vi "TrALEX_NRG.vi"(0 "Analog Amplitude":dbl=1.0 format="%0.2p", 1 "Repetition Frequency":dbl=2.0 format="%.6f") -> ()   [LabVIEW 2011]
uses:
  <vilib>/DAQmx/write.llb/DAQmx Write (Analog Wfm 1Chan NSamp).vi
  <vilib>/DAQmx/create/channels.llb/DAQmx Create Channel (AO-Voltage-Basic).vi
  <vilib>/DAQmx/configure/timing.llb/DAQmx Timing (Sample Clock).vi
  <vilib>/DAQmx/create/channels.llb/DAQmx Create Channel (CO-Pulse Generation-Frequency).vi
  <vilib>/DAQmx/configure/events/hardwareSignals.llb/DAQmx Export Signal (Most Signals).vi
  <vilib>/DAQmx/configure/trigger.llb/DAQmx Start Trigger (Digital Edge).vi
  <vilib>/DAQmx/configure/timing.llb/DAQmx Timing (Implicit).vi
  <vilib>/DAQmx/miscellaneous.llb/DAQmx Fill In Error Info.vi
  <vilib>/measure/NI_MABase.lvlib
panel:
  in  "Three Colour Duty Cycle":dbl=0.3333333333333333 format="%.6f"
  in  "Stop Button":bool
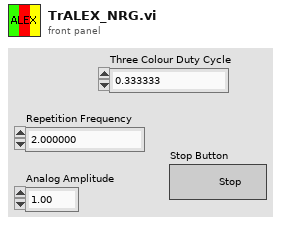
[diagram p1: front panel]
types:
  T1 = enum16{"Sine Wave", "Triangle Wave", "Square Wave", "Sawtooth Wave"}
  T2 = cluster{"Ao0 Sample Clock Rate":dbl, "Ao0 Sample Clock Rate":dbl}
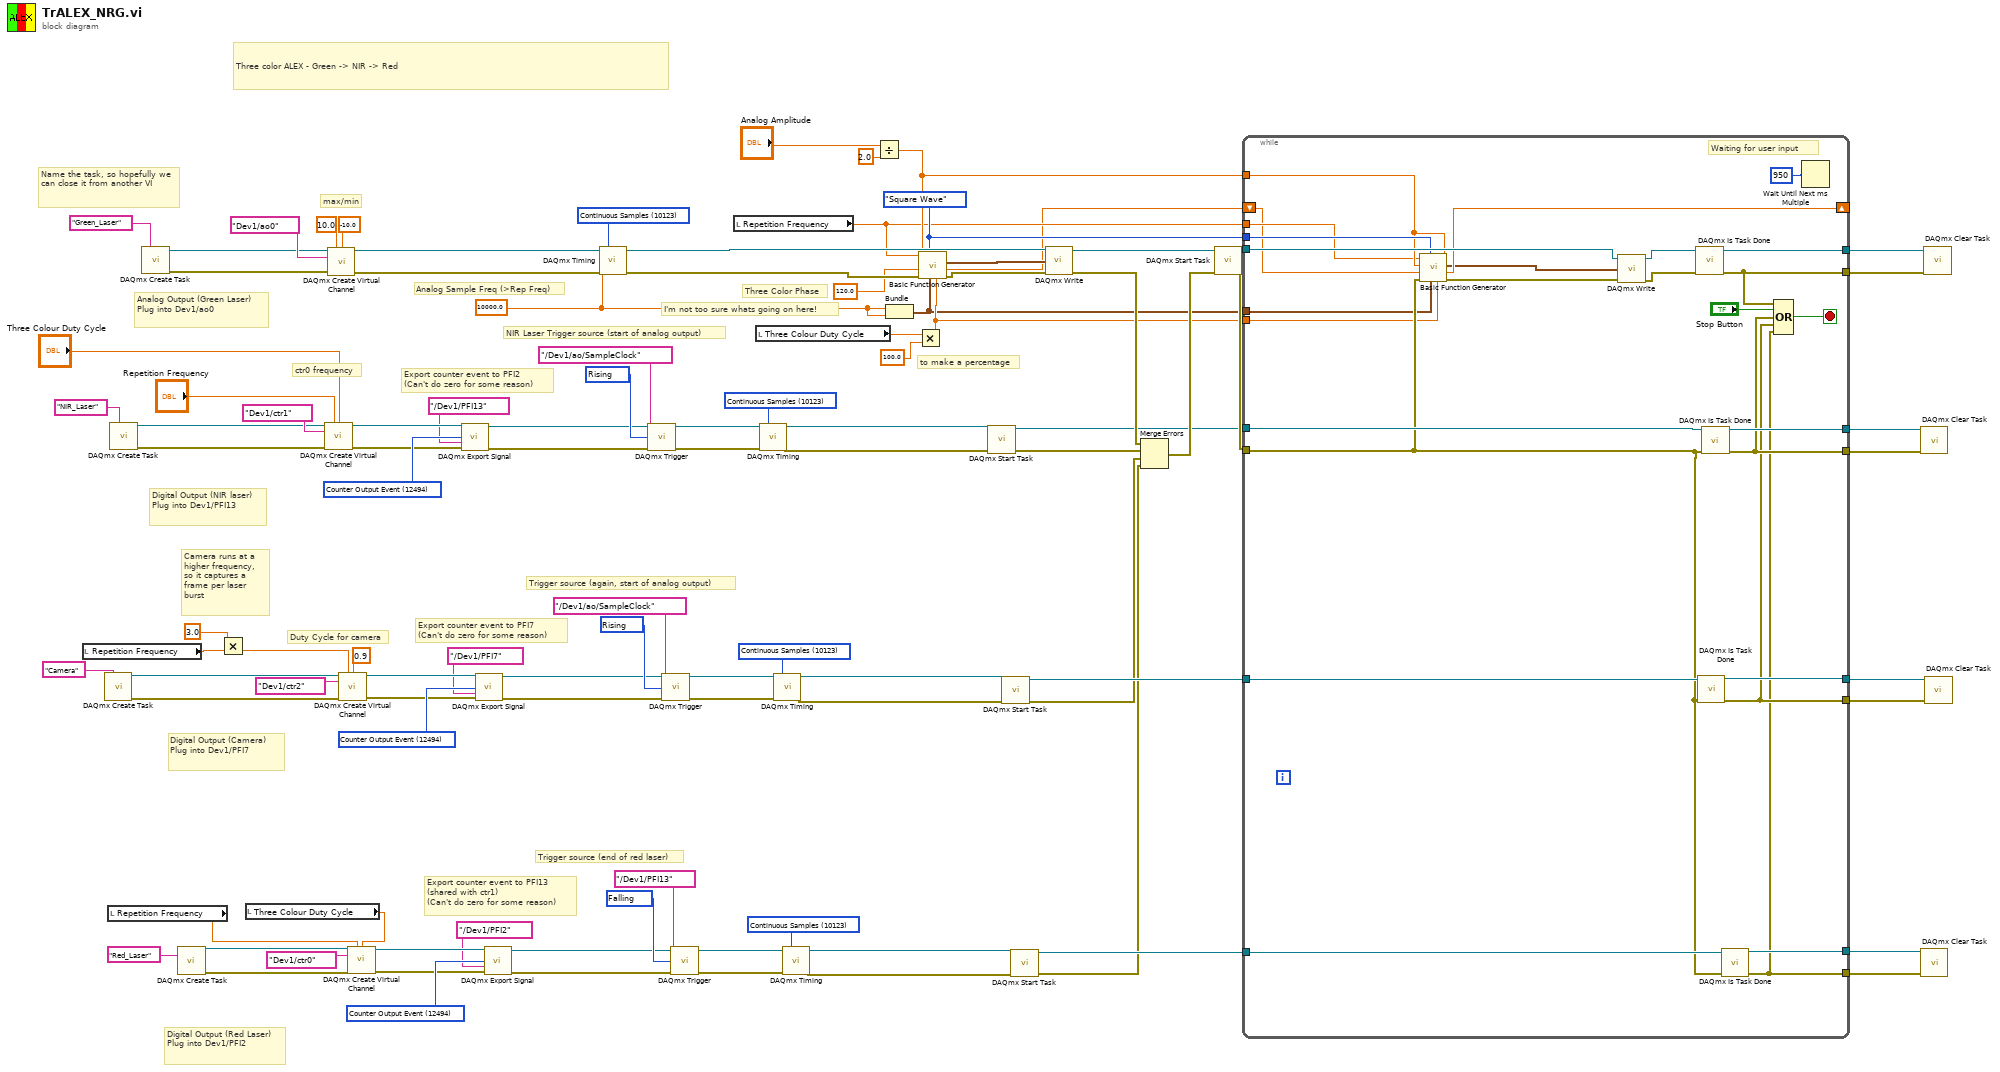
[diagram p0: block diagram]
diagram:
  w35 = 10171 items=["Rising"=10280, "Falling"=10171] ("edge")
  w38 = 10123 items=["Finite Samples"=10178, "Continuous Samples"=10123, "Hardware Timed Single Point"=12522] ("sample mode")
  w40 = 12494 items=["AI Convert Clock"=12484, "10MHz Reference Clock"=12536, "20MHz Timebase Clock"=12486, "Sample Clock"=12487, "Advance Trigger"=12488, "Reference Trigger"=12490, "Start Trigger"=12491, "Advance Complete Event"=12492, "AI Hold Complete Event"=12493, "Counter Output Event"=12494, "Change Detection Event"=12511, "Watchdog Timer Expired Event"=12512] ("signal")
  w58 = 10280 items=["Rising"=10280, "Falling"=10171] ("edge")
  w61 = 10123 items=["Finite Samples"=10178, "Continuous Samples"=10123, "Hardware Timed Single Point"=12522] ("sample mode")
  w63 = 12494 items=["AI Convert Clock"=12484, "10MHz Reference Clock"=12536, "20MHz Timebase Clock"=12486, "Sample Clock"=12487, "Advance Trigger"=12488, "Reference Trigger"=12490, "Start Trigger"=12491, "Advance Complete Event"=12492, "AI Hold Complete Event"=12493, "Counter Output Event"=12494, "Change Detection Event"=12511, "Watchdog Timer Expired Event"=12512] ("signal")
  w70 = 10123 items=["Finite Samples"=10178, "Continuous Samples"=10123, "Hardware Timed Single Point"=12522] ("sample mode")
  w5 = T1."Square Wave" ("signal type")
  w90 = 10280 items=["Rising"=10280, "Falling"=10171] ("edge")
  w95 = 10123 items=["Finite Samples"=10178, "Continuous Samples"=10123, "Hardware Timed Single Point"=12522] ("sample mode")
  w97 = 12494 items=["AI Convert Clock"=12484, "10MHz Reference Clock"=12536, "20MHz Timebase Clock"=12486, "Sample Clock"=12487, "Advance Trigger"=12488, "Reference Trigger"=12490, "Start Trigger"=12491, "Advance Complete Event"=12492, "AI Hold Complete Event"=12493, "Counter Output Event"=12494, "Change Detection Event"=12511, "Watchdog Timer Expired Event"=12512] ("signal")
  w42 = 10000.0 ("Ao0 Sample Clock Rate")
  # "Three color ALEX - Green -> NIR -> Red"
  # "Name the task, so hopefully we can close it from another VI"
  # "to make a percentage"
  # "Digital Output (Red Laser) Plug into Dev1/PFI2"
  # "Trigger source (end of red laser)"
  # "Export counter event to PFI13 (shared with ctr1)\n(Can't do zero for some reason)"
  # "Duty Cycle for camera"
  # "Camera runs at a higher frequency, so it captures a frame per laser burst"
  # "Digital Output (Camera) Plug into Dev1/PFI7"
  # "Trigger source (again, start of analog output)"
  # "Export counter event to PFI7\n(Can't do zero for some reason)"
  # "Digital Output (NIR laser) Plug into Dev1/PFI13"
  # "Analog Output (Green Laser) Plug into Dev1/ao0"
  # "Three Color Phase"
  # "Analog Sample Freq (>Rep Freq)"
  # "I'm not too sure whats going on here!"
  # "NIR Laser Trigger source (start of analog output)"
  # "Export counter event to PFI2\n(Can't do zero for some reason)"
  # "ctr0 frequency"
  # "max/min"
  n1 = local read "Repetition Frequency"() -> (w50:dbl)
  n2 = call <vilib>:"DAQmx Create Task.vi"("new task name"="Camera") -> ("task out"=w10:refnum<k21>, "error out"=w9:errorcluster)  [unwired: 13 in]
  n3 = local read "Repetition Frequency"() -> (w20:dbl)
  n4 = call <vilib>:"DAQmx Create Task.vi"("new task name"="NIR_Laser") -> ("task out"=w12:refnum<k21>, "error out"=w11:errorcluster)  [unwired: 13 in]
  n5 = call <vilib>:"DAQmx Create Task.vi"("new task name"="Green_Laser") -> ("task out"=w18:refnum<k21>, "error out"=w17:errorcluster)  [unwired: 13 in]
  n6 = call <vilib>:"DAQmx Create Task.vi"("new task name"="Red_Laser") -> ("task out"=w8:refnum<k21>, "error out"=w7:errorcluster)  [unwired: 13 in]
  n7 = Multiply(x=3.0 ("Repetition Frequency"), y=w50) -> (x*y=w49:dbl)
  n8 = local read "Three Colour Duty Cycle"() -> (w24:dbl)
  n9 = call-poly <vilib>:"DAQmx Create Virtual Channel.vi"("task in"=w12, "frequency"="Repetition Frequency", "duty cycle"="Three Colour Duty Cycle", "counter"=tag "Dev1/ctr1", "error in"=w11) -> ("task out"=w98:refnum<k21>, "error out"=w96:errorcluster)  [unwired: 9 in]
  n10 = call-poly <vilib>:"DAQmx Create Virtual Channel.vi"("task in"=w18, "maximum value"=10.0, "minimum value"=-10.0, "physical channels"=tag "Dev1/ao0", "error in"=w17) -> ("task out"=w102:refnum<k21>, "error out"=w101:errorcluster)  [unwired: 9 in]
  n11 = call-poly <vilib>:"DAQmx Create Virtual Channel.vi"("task in"=w10, "frequency"=w49, "duty cycle"=0.9, "counter"=tag "Dev1/ctr2", "error in"=w9) -> ("task out"=w64:refnum<k21>, "error out"=w62:errorcluster)  [unwired: 9 in]
  n12 = call-poly <vilib>:"DAQmx Create Virtual Channel.vi"("task in"=w8, "frequency"=w20, "duty cycle"=w24, "counter"=tag "Dev1/ctr0", "error in"=w7) -> ("task out"=w41:refnum<k21>, "error out"=w39:errorcluster)  [unwired: 9 in]
  n13 = call-poly <vilib>:"DAQmx Export Signal.vi"("task/channels in"=w98, "signal"=w97, "output terminal"=tag "/Dev1/PFI13", "error in"=w96) -> ("task out"=w89:refnum<k21>, "error out"=w86:errorcluster)  [unwired: 10 in]
  n14 = call-poly <vilib>:"DAQmx Export Signal.vi"("task/channels in"=w64, "signal"=w63, "output terminal"=tag "/Dev1/PFI7", "error in"=w62) -> ("task out"=w57:refnum<k21>, "error out"=w54:errorcluster)  [unwired: 10 in]
  n15 = call-poly <vilib>:"DAQmx Export Signal.vi"("task/channels in"=w41, "signal"=w40, "output terminal"=tag "/Dev1/PFI2", "error in"=w39) -> ("task out"=w34:refnum<k21>, "error out"=w31:errorcluster)  [unwired: 10 in]
  n16 = call-poly <vilib>:"DAQmx Timing.vi"("task/channels in"=w102, "sample mode"=w70, "rate"=w42, "error in"=w101) -> ("task out"=w94:refnum<k21>, "error out"=w93:errorcluster)  [unwired: 10 in]
  n17 = call-poly <vilib>:"DAQmx Trigger.vi"("task/channels in"=w89, "source"=tag "/Dev1/ao/SampleClock", "edge"=w90, "error in"=w86) -> ("task out"=w88:refnum<k21>, "error out"=w87:errorcluster)  [unwired: 10 in]
  n18 = call-poly <vilib>:"DAQmx Trigger.vi"("task/channels in"=w57, "source"=tag "/Dev1/ao/SampleClock", "edge"=w58, "error in"=w54) -> ("task out"=w56:refnum<k21>, "error out"=w55:errorcluster)  [unwired: 10 in]
  n19 = call-poly <vilib>:"DAQmx Trigger.vi"("task/channels in"=w34, "source"=tag "/Dev1/PFI13", "edge"=w35, "error in"=w31) -> ("task out"=w33:refnum<k21>, "error out"=w32:errorcluster)  [unwired: 10 in]
  n20 = local read "Repetition Frequency"() -> (w4:dbl)
  n21 = local read "Three Colour Duty Cycle"() -> (w26:dbl)
  n22 = call-poly <vilib>:"DAQmx Timing.vi"("task/channels in"=w88, "sample mode"=w95, "error in"=w87) -> ("task out"=w83:refnum<k21>, "error out"=w82:errorcluster)  [unwired: 11 in]
  n23 = call-poly <vilib>:"DAQmx Timing.vi"("task/channels in"=w56, "sample mode"=w61, "error in"=w55) -> ("task out"=w53:refnum<k21>, "error out"=w52:errorcluster)  [unwired: 11 in]
  n24 = call-poly <vilib>:"DAQmx Timing.vi"("task/channels in"=w33, "sample mode"=w38, "error in"=w32) -> ("task out"=w30:refnum<k21>, "error out"=w29:errorcluster)  [unwired: 11 in]
  n25 = Divide(x="Analog Amplitude", y=2.0) -> (x/y=w6:dbl)
  n26 = Bundle("Ao0 Sample Clock Rate"=w42, "Ao0 Sample Clock Rate"=w42) -> (w1:T2)  [unwired: 1 in]
  n27 = Multiply(x=w26, y=100.0) -> (x*y=w2:dbl)
  n28 = call <vilib>:"Basic Function Generator.vi"("offset"=w6, "square wave duty cycle (%)"=w2, "sampling info"=w1, "signal type"=w5, "error in (no error)"=w93, "phase"=120.0, "amplitude"=w6, "frequency"=w4) -> ("error out"=w84:errorcluster, "phase out"=w3:dbl, "signal out"=w85:waveform(dbl))  [unwired: 1 in]
  n29 = call <vilib>:"DAQmx Start Task.vi"("task/channels in"=w83, "error in"=w82) -> ("task out"=w71:refnum<k21>, "error out"=w81:errorcluster)  [unwired: 12 in]
  n30 = call <vilib>:"DAQmx Start Task.vi"("task/channels in"=w53, "error in"=w52) -> ("task out"=w46:refnum<k21>, "error out"=w45:errorcluster)  [unwired: 12 in]
  n31 = call <vilib>:"DAQmx Start Task.vi"("task/channels in"=w30, "error in"=w29) -> ("task out"=w23:refnum<k21>, "error out"=w19:errorcluster)  [unwired: 12 in]
  n32 = call-poly <vilib>:"DAQmx Write.vi"("task/channels in"=w94, "data"=w85, "error in"=w84) -> ("task out"=w78:refnum<k21>, "error out"=w80:errorcluster)  [unwired: 10 in, 1 out]
  n33 = Merge Errors(w80, w81, w45, w19) -> (w79:errorcluster)
  n34 = call <vilib>:"DAQmx Start Task.vi"("task/channels in"=w78, "error in"=w79) -> ("task out"=w77:refnum<k21>, "error out"=w76:errorcluster)  [unwired: 12 in]
  n35 = while {
    tunnel: [w130] -> w72
    tunnel: [w124] -> w75
    tunnel: [w127] -> w73
    tunnel: [w122] -> w74
    tunnel: w77 -> [w114]
    tunnel: w76 -> [w108]
    tunnel: w71 -> [w126]
    tunnel: w46 -> [w125]
    tunnel: [w121] -> w44
    tunnel: [w120] -> w43
    tunnel: w23 -> [w119]
    tunnel: [w118] -> w22
    tunnel: [w117] -> w21
    tunnel: w6 -> [w112]
    tunnel: w5 -> [w113]
    tunnel: w4 -> [w111]
    shift-right: [w110] -> _
    shift-left: w3 -> [w109]
    tunnel: w2 -> [w107]
    tunnel: w1 -> [w106]
    stop <- w128 stop-if-true
    # "Waiting for user input"
    n36 = call <vilib>:"Basic Function Generator.vi"("offset"=w112, "square wave duty cycle (%)"=w107, "sampling info"=w106, "signal type"=w113, "error in (no error)"=w108, "phase"=w109, "amplitude"=w112, "frequency"=w111) -> ("error out"=w105:errorcluster, "phase out"=w110:dbl, "signal out"=w104:waveform(dbl))  [unwired: 1 in]
    n37 = call-poly <vilib>:"DAQmx Write.vi"("task/channels in"=w114, "data"=w104, "error in"=w105) -> ("task out"=w116:refnum<k21>, "error out"=w115:errorcluster)  [unwired: 10 in, 1 out]
    n38 = call <vilib>:"DAQmx Is Task Done.vi"("task/channels in"=w116, "error in"=w115) -> ("task out"=w130:refnum<k21>, "error out"=w124:errorcluster)  [unwired: 11 in, 1 out]
    n39 = call <vilib>:"DAQmx Is Task Done.vi"("task/channels in"=w125, "error in"=w108) -> ("task out"=w121:refnum<k21>, "error out"=w120:errorcluster)  [unwired: 11 in, 1 out]
    n40 = call <vilib>:"DAQmx Is Task Done.vi"("task/channels in"=w126, "error in"=w108) -> ("task out"=w127:refnum<k21>, "error out"=w122:errorcluster)  [unwired: 11 in, 1 out]
    n41 = call <vilib>:"DAQmx Is Task Done.vi"("task/channels in"=w119, "error in"=w108) -> ("task out"=w118:refnum<k21>, "error out"=w117:errorcluster)  [unwired: 11 in, 1 out]
    n42 = Compound Arithmetic op=OR(w124, "Stop Button", w122, w120, w117) -> (w128:bool)
    n43 = Wait Until Next ms Multiple(millisecond multiple=u32 950) -> ()  [unwired: 1 out]
  }
  n44 = call <vilib>:"DAQmx Clear Task.vi"("task in"=w73, "error in"=w74) -> ()  [unwired: 13 in, 1 out]
  n45 = call <vilib>:"DAQmx Clear Task.vi"("task in"=w22, "error in"=w21) -> ()  [unwired: 13 in, 1 out]
  n46 = call <vilib>:"DAQmx Clear Task.vi"("task in"=w72, "error in"=w75) -> ()  [unwired: 13 in, 1 out]
  n47 = call <vilib>:"DAQmx Clear Task.vi"("task in"=w44, "error in"=w43) -> ()  [unwired: 13 in, 1 out]
